vi "TEST - Reshape Array to 1D VArray.vi"(8 "error in (no error)":errorcluster) -> (0 "error out":errorcluster, 2 "pass":bool)   [LabVIEW 2020, in "test_openg_variant.lvlib"]
uses:
  test_openg_variant.lvlib
  <userlib>/_OpenG.lib/error/error.llb/openg_error.lvlib
  source/library/openg_variant.lvlib
panel:
  out "Failures":T1(array[cluster])
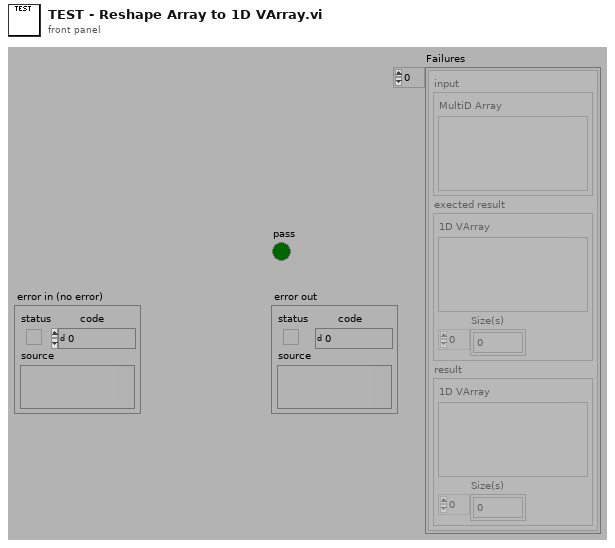
[diagram p1: front panel]
types:
  T1 = cluster{"input":cluster{"MultiD Array":variant}, "exected result":cluster{"1D VArray":variant, "Size(s)":u32[]}, "result":cluster{"1D VArray":variant, "Size(s)":u32[]}}[]
  T2 = cluster{"input":cluster{"MultiD Array":variant}, "exected result":cluster{"1D VArray":variant, "Size(s)":u32[]}, "result":cluster{"1D VArray":variant, "Size(s)":u32[]}}
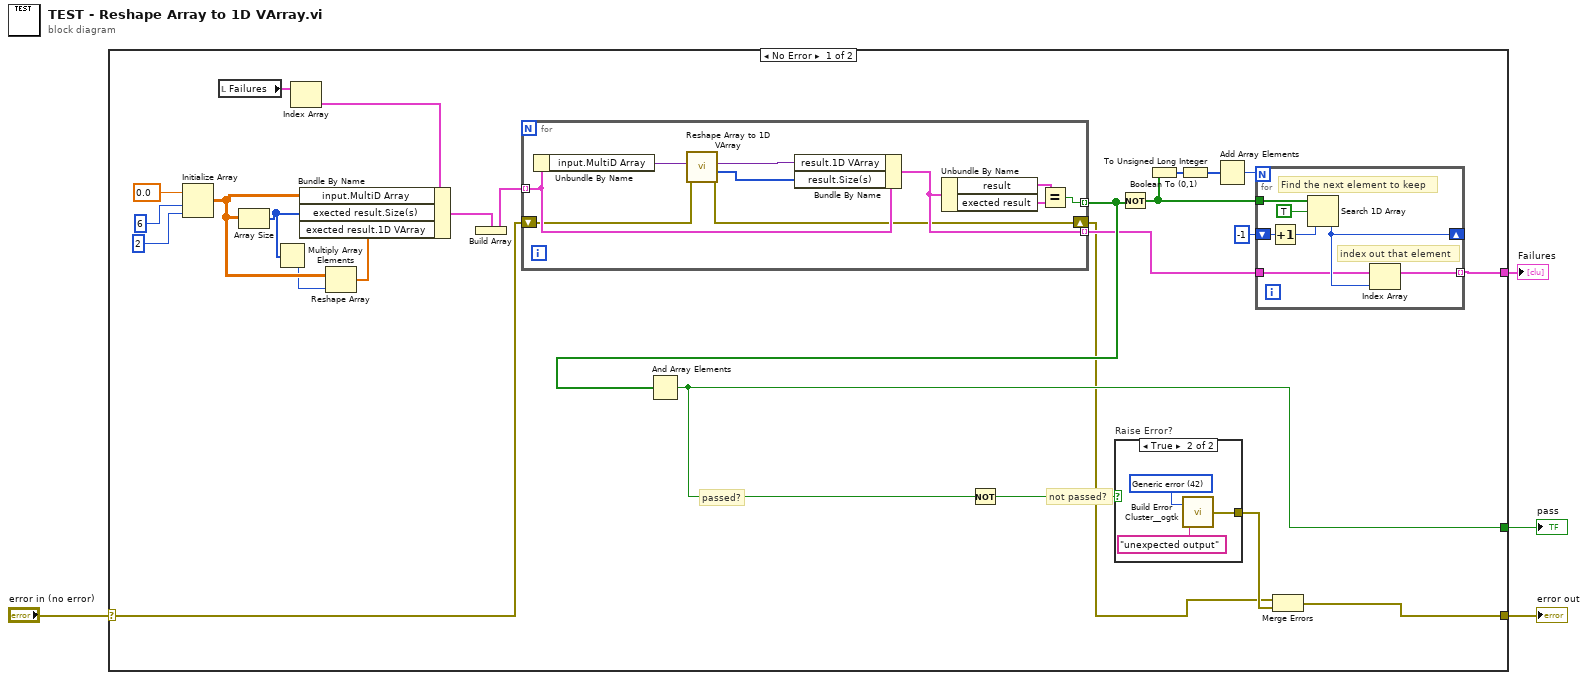
[diagram p0: block diagram]
diagram:
  n1 = case shown="No Error" "error in (no error)" {
    selector: "error in (no error)" -> [w15 w50]
    tunnel: [w26 _] -> w4
    tunnel: [w29 w50] -> w2
    tunnel: [w18 _] -> w1
    frame No Error {
      # "not passed?"
      # "passed?"
      n2 = Initialize Array(0.0 ("element"), 6 ("dimension size"), 2 ("dimension size")) -> (w8:dbl[][])
      n3 = local read "Failures"() -> (w13:T1)
      n4 = Array Size(array=w8) -> (size(s)=w7:i32[])
      n5 = Multiply Array Elements(1:w7) -> (0:w6:i32)
      n6 = Index Array(array=w13) -> (element=w12:T2)  [unwired: 1 in]
      n7 = Reshape Array(w8, w6) -> (w5:dbl[])
      n8 = Bundle By Name(cluster=w12, "input.MultiD Array"=w8, "exected result.Size(s)"=w7, "exected result.1D VArray"=w5) -> (w17:T2)
      n9 = Build Array(w17) -> (w16:T1)
      n10 = for {
        tunnel: w16 -> [w45] mode=indexing
        tunnel: [w46] -> w20 mode=indexing
        tunnel: [w44] -> w19 mode=indexing
        shift-right: [w40] -> w14
        shift-left: w15 -> [w39]
        n11 = Unbundle By Name(w45) -> ("input.MultiD Array"=w41:variant)
        n12 = call "Reshape Array to 1D VArray.vi"("error in (no error)"=w39, "MultiD Array"=w41) -> ("error out"=w40:errorcluster, "Size(s)"=w37:u32[], "1D VArray"=w38:variant)  [unwired: 7 in]
        n13 = Bundle By Name(cluster=w45, "result.1D VArray"=w38, "result.Size(s)"=w37) -> (w44:T2)
        n14 = Unbundle By Name(w44) -> ("result"=w43:cluster{"1D VArray":variant, "Size(s)":u32[]}, "exected result"=w42:cluster{"1D VArray":variant, "Size(s)":u32[]})
        n15 = Equal?(x=w43, y=w42) -> (x = y?=w46:bool)
      }
      n16 = And Array Elements(Boolean array=w20) -> (logical AND=w26:bool)
      n17 = Not(x=w26) -> (.not. x?=w27:bool)
      n18 = case "Raise Error?" shown="True" w27 {
        tunnel: [_ w47] -> w28
        frame False {
        }
        frame True {
          w48 = 42 items=["No error", "Argument error", "Memory is full", "Out of zone", "End of file", "File already open", "Generic file I/O error", "File not found", "File permission error", "Disk is full", "Duplicate path", "Too many files open", "System feature not enabled", "Resource file not found", "Cannot add resource", "Resource not found", "Image not found", "Image memory error", "Pen does not exist", "Config type invalid", "Config token not found", "Config parse error", "Config memory error", "Bad external code format", "Bad external code offset", "External code not present", "Null window", "Destroy window error", "Null menu", "Print aborted", "Bad print record", "Print driver error", "Windows error during printing", "Memory error during printing", "Print dialog error", "Generic print error", "Invalid device refnum", "Device not found", "Device parameter error", "Device unit error", "Cannot open device", "Device call aborted", "Generic error", "Cancelled by user", "Object ID too low", "Object ID too high", "Object not in heap", "Unknown heap", "Unknown object (invalid DefProc)", "Unknown object (DefProc not in table)", "Message out of range", "Invalid (null) method", "Unknown message", "Manager call not supported", "Bad address", "Network operation in progress", "Network operation timed out", "Connection is busy", "Network attribute not supported", "Network error", "Address in use", "System out of memory", "Connection aborted", "Connection refused", "Not connected", "Already connected", "Connection closed", "Initialization error (interapplication manager)", "Bad occurrence", "Wait on unbound occurrence handler", "Occurrence queue overflow", "Datalog type conflict", "Unused", "Unrecognized type (interapplication manager)", "Memory corrupt", "Failed to make temporary DLL", "Old CIN version", "Drag socket not found", "Failed to load drop-object", "Failed to register OLE object", "Failed to release OLE object", "Format specifier type mismatch", "Unknown format specifier", "Too few format specifiers", "Too many format specifiers", "Scan failed", "Newer CIN version", "Error converting to variant", "Runtime menu error", "Password tampered", "Variant attribute not found", "Incompatible variant data type", "Event data is not available", "Event Store is not present", "Occurrence is not found", "Event Queue is not created", "Event info is not available", "Refnum passed is NULL", "Error retrieving Class GUID", "Error retrieving CoClass GUID", "Error retrieving TypeLib GUID.", "Bad built application magic bytes.", "Specific driver is different from the specific driver associated with the Logical Name.", "There is no session opened to the class driver.", "Max Error", "MAX - Error with config objects", "MAX - Error loading configuration", "MAX - Group not supported"]
          n19 = call <userlib>:"Build Error Cluster__ogtk.vi"("String to Prepend to source (\"\")"="unexpected output" ("String to Prepend to source (\"\")"), "code"=w48) -> ("error out"=w47:errorcluster)
        }
      }
      n20 = Not(x=w20) -> (.not. x?=w22:bool[])
      n21 = Boolean To (0,1)(Boolean=w22) -> (0, 1=w23:i16[])
      n22 = To Unsigned Long Integer(number=w23) -> (unsigned 32bit integer=w21:u32[])
      n23 = Add Array Elements(numeric array=w21) -> (sum=w24:u32)
      n24 = for {
        N: w24 -> [_]
        tunnel: w19 -> [w32]
        tunnel: w22 -> [w36]
        shift-right: [w33] -> _
        shift-left: -1 ("start index (0)") -> [w34]
        tunnel: [w31] -> w18 mode=indexing
        # "index out that element"
        # "Find the next element to keep"
        n25 = Increment(x=w34) -> (x+1=w30:i32)
        n26 = Search 1D Array(1D array=w36, element=TRUE, start index (0)=w30) -> (index of element=w33:i32)
        n27 = Index Array(array=w32, index=w33) -> (element=w31:T2)
      }
      n28 = Merge Errors(w14, w28) -> (w29:errorcluster)
    }
    frame Error {
    }
  }
  "pass" <- w4
  "error out" <- w2
  "Failures" <- w1
